vi "DeleteVarFromGroup.vi"(8 "error in (no error)":errorcluster, 10 "VariableName":string, 11 "VariableGroup in":refnum<class "VariableGroup.lvclass">) -> (0 "error out":errorcluster, 3 "VariableGroup out":refnum<class "VariableGroup.lvclass">)   [LabVIEW 2013, in "VariableGroup.lvclass"]
doc: "Remove VariableName from DisplayList of the VariableGroup.\nNo operation if there is no VariableName in the DisplayList of the VariableGroup."
uses:
  VariableGroup.lvclass
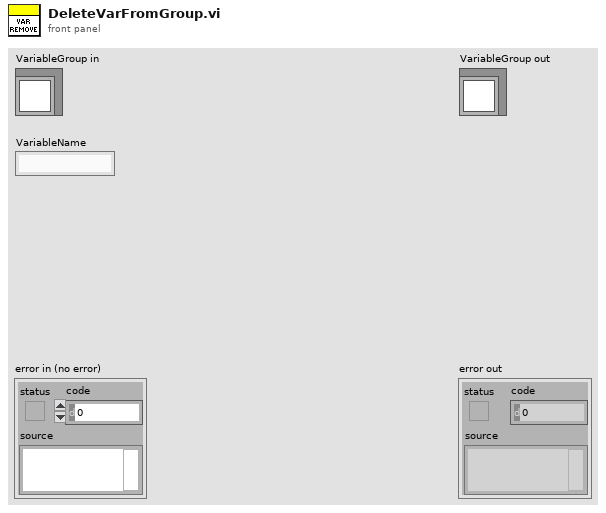
[diagram p1: front panel]
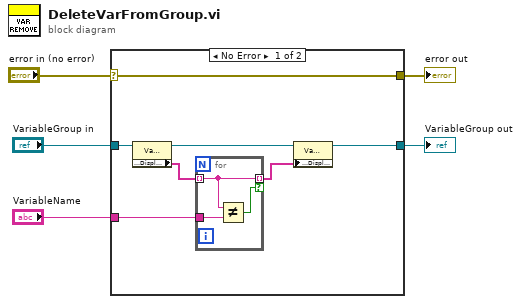
[diagram p0: block diagram]
diagram:
  n1 = case shown="No Error" "error in (no error)" {
    selector: "error in (no error)" -> [w12 w17]
    tunnel: [w12 w17] -> w4
    tunnel: [w6 w16] -> w2
    tunnel: "VariableGroup in" -> [w9 w16]
    tunnel: "VariableName" -> [w11 _]
    frame No Error {
      n2 = property class="VariableGroup.lvclass"(reference=w9) -> (reference out=w8:refnum<class "VariableGroup.lvclass">, "Accessors:DisplayList"=w10:string[])  [unwired: 1 in, 1 out]
      n3 = for {
        tunnel: w10 -> [w14] mode=indexing
        tunnel: [w14] -> w7 mode=indexing if=w15
        tunnel: w11 -> [w13]
        n4 = Not Equal?(x=w14, y=w13) -> (x != y?=w15:bool)
      }
      n5 = property class="VariableGroup.lvclass"(reference=w8, "Accessors:DisplayList"=w7) -> (reference out=w6:refnum<class "VariableGroup.lvclass">)  [unwired: 1 in, 1 out]
    }
    frame Error {
    }
  }
  "error out" <- w4
  "VariableGroup out" <- w2
